vi "NA  DB Cluster v1_0_0.vi"() -> (0 "FVP  MAIN":T3={"general"={"project directory"=path "C:/NA", "User Name"="", "User Level"="", "valid login"=TRUE, "screen size"=1, "Screen Width"=1, "Screen Height"=1, "Login Password"="", "Login User Name"="", ".ini Resources"=[], "Control Refs"=[], "Error Ref out"=refnum, "DB Ref"=refnum}, "rendezvous"=refnum, "queues"={"Main"=refnum, "Error"=refnum, "DAQ"=refnum, "VFP"=refnum}, "NI Testand Config"={"NI_Teststand DB"=[]}, "Test Station Config"={"Test Station DB"=[], "Button Names"=[], "Short-cut keys"=[], "Paths to vis"=[], "Sub-Panel"=[], "Wait until done"=[], "Delay"=[], "Dispose Ref"=[], "Var. 1"=[], "Var. 2"=[], "Descriptions"=[], "Show Button"=[], "Short-cut from DB"=[], "Prefix"=[]}, "Sub Panel"={"Position"={"Left"=0, "Top"=0}, "Hidden Pos"={"Left"=0, "Top"=0}}})   [LabVIEW 2009]
doc: "WGLOV Cluster v1_0_0.vi\n\n\nGeneral Cluster constant used for start of state machine templates"
uses:
  <vilib>/addons/database/Connection.llb/Conn ObjectReference.ctl
  <vilib>/addons/database/NI_Database_API.lvlib
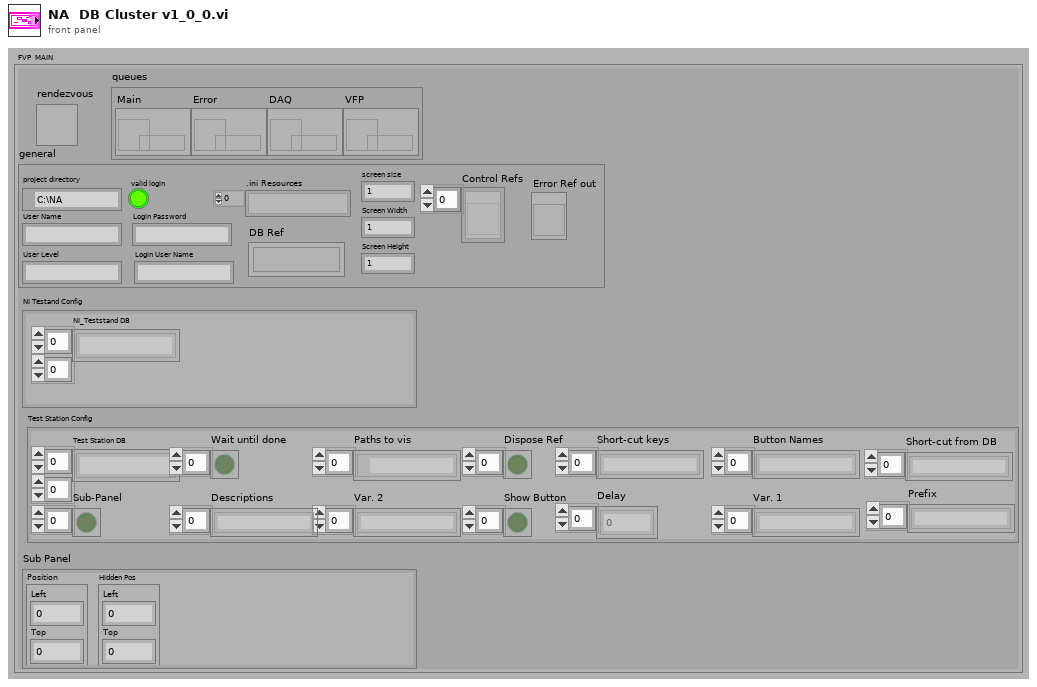
[diagram p1: front panel]
types:
  T1 = typedef "NI_Database_API.lvlib/Conn ObjectReference.ctl" = refnum<k1>
  T2 = typedef "Rendezvous RefNum" = refnum<k1>
  T3 = cluster{"general":cluster{"project directory":path, "User Name":string, "User Level":string, "valid login":bool, "screen size":i32, "Screen Width":i32, "Screen Height":i32, "Login Password":string, "Login User Name":string, ".ini Resources":string[], "Control Refs":refnum<vi>[], "Error Ref out":refnum<vi>, "DB Ref":T1}, "rendezvous":T2, "queues":cluster{"Main":refnum<queue>, "Error":refnum<queue>, "DAQ":refnum<queue>, "VFP":refnum<queue>}, "NI Testand Config":cluster{"NI_Teststand DB":string[][]}, "Test Station Config":cluster{"Test Station DB":string[][], "Button Names":string[], "Short-cut keys":string[], "Paths to vis":path[], "Sub-Panel":bool[], "Wait until done":bool[], "Delay":i32[], "Dispose Ref":bool[], "Var. 1":string[], "Var. 2":string[], "Descriptions":string[], "Show Button":bool[], "Short-cut from DB":string[], "Prefix":string[]}, "Sub Panel":cluster{"Position":cluster{"Left":i32, "Top":i32}, "Hidden Pos":cluster{"Left":i32, "Top":i32}}}
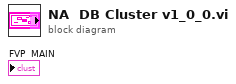
[diagram p0: block diagram]
diagram:
